vi "subStage_Initialize.vi"(7 "Stage setting":T3={"Baudrate"=57600, "COM Port"="COM10", "Xmax"=118.5, "Xmin"=15.0, "Ymax"=76.5, "Ymin"=12.2}, 8 "Error In":errorcluster, 11 "Stage-Ctrl":T1={"Console"={"L"=FALSE, "R"=FALSE, "FWD"=FALSE, "BACK"=FALSE}, "Step Width [mm]"=1.0, "Destination [mm]"=[1.02, -2.92], "Move "=FALSE} {"Destination [mm]" format="%_6g"; "Step Width [mm]" min=0.0 format="%_6f"}) -> (0 "Error out":errorcluster, 3 "Stage initialized":bool=TRUE, 5 "Stage Info":T2={" Current Position"=[-1.0, -12.0, 0.0], "Number of Axis"=3, "ILSID"=1})   [LabVIEW 2015]
panel:
  # "X"
  # "Y"
  # "X"
  # "Y"
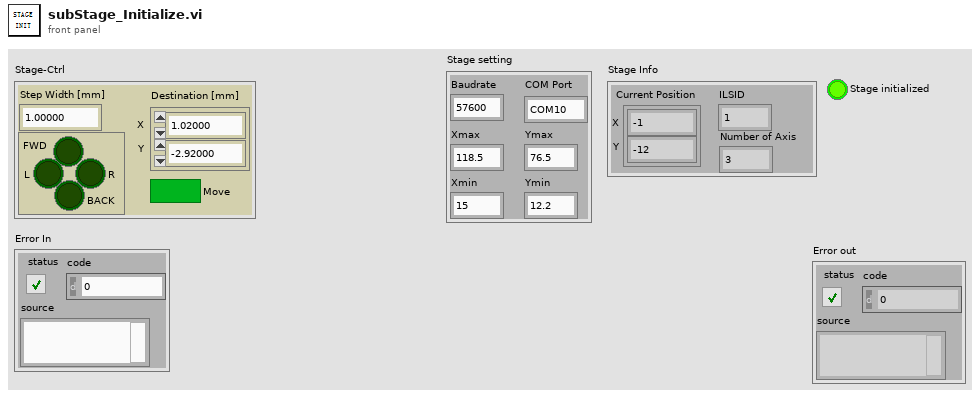
[diagram p1: front panel]
types:
  T1 = cluster{"Console":cluster{"L":bool, "R":bool, "FWD":bool, "BACK":bool}, "Step Width [mm]":dbl, "Destination [mm]":dbl[], "Move ":bool}
  T2 = cluster{" Current Position":dbl[], "Number of Axis":i32, "ILSID":i32}
  T3 = cluster{"Baudrate":i32, "COM Port":string, "Xmax":dbl, "Xmin":dbl, "Ymax":dbl, "Ymin":dbl}
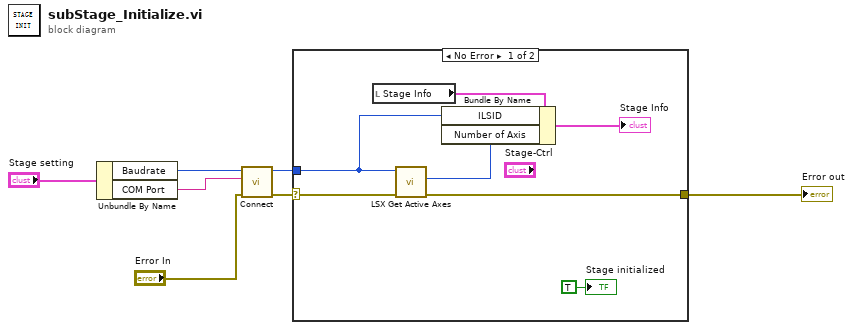
[diagram p0: block diagram]
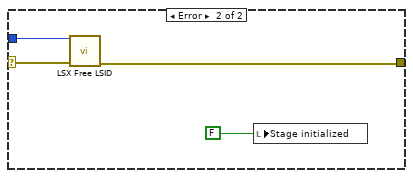
[diagram p2: hidden frame]
diagram:
  n1 = Unbundle By Name("Stage setting") -> ("Baudrate"=w5:i32, "COM Port"=w6:string)
  n2 = call "Connect.vi"("error in (no error)"="Error In", "pcAComName"=w6, "lABaudRate"=w5) -> ("error out"=w2:errorcluster, "plLSID out"=w4:i32)  [unwired: 5 in, 1 out]
  n3 = case shown="No Error" w2 {
    selector: w2 -> [w14 w18]
    tunnel: w4 -> [w12 w16]
    tunnel: [w9 w17] -> w1
    frame No Error {
      n4 = local read "Stage Info"() -> (w13:T2)
      n5 = call <userlib>:"LSX Get Active Axes.vi"("error in (no error)"=w14, "lLSID"=w12) -> ("error out"=w9:errorcluster, "plFlags out"=w11:i32)  [unwired: 7 in, 1 out]
      n6 = Bundle By Name(cluster=w13, "ILSID"=w12, "Number of Axis"=w11) -> (→"Stage Info":T2)
      "Stage initialized" <- TRUE ("Stage initialized")
    }
    frame Error {
      n7 = call <userlib>:"LSX Free LSID.vi"("error in (no error)"=w18, "lLSID"=w16) -> ("error out"=w17:errorcluster)  [unwired: 8 in, 1 out]
      n8 = local write "Stage initialized"(FALSE ("Stage initialized")) -> ()
    }
  }
  "Error out" <- w1
